vi "sub_Mock_system_IO.vi"(5 "error in":errorcluster) -> (0 "error out":errorcluster, 1 "rate":dbl=25600.0, 2 "displacement task":refnum<k21>)   [LabVIEW 2019]
uses:
  <vilib>/DAQmx/create/channels.llb/DAQmx Create Channel (AI-Voltage-Basic).vi
  <vilib>/DAQmx/configure/timing.llb/DAQmx Timing (Sample Clock).vi
  <resource>/objmgr/daqmx.rc
  <vilib>/DAQmx/write.llb/DAQmx Write (Digital 1D Bool NChan 1Samp 1Line).vi
  <vilib>/DAQmx/create/channels.llb/DAQmx Create Channel (DO-Digital Output).vi
  <vilib>/DAQmx/create/channels.llb/DAQmx Create Channel (AI-Acceleration-Accelerometer).vi
  <vilib>/DAQmx/read.llb/DAQmx Read (Analog 1D DBL 1Chan NSamp).vi
panel:
  out "time ACC Data collection":dbl
  out "acc error":errorcluster
  out "acc task":refnum<k21>
  out "Accel Data":dbl[](array[numeric])
  out "error out parker":errorcluster
  out "Parker task":refnum<k21>
  out "accelerometer sample rate (S/s)":dbl
  in  "parker error in (no error)":errorcluster caption="error in (no error)"
  in  "error in 2":errorcluster caption="error in"
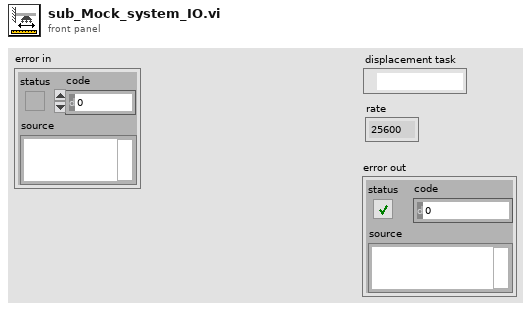
[diagram p1: front panel]
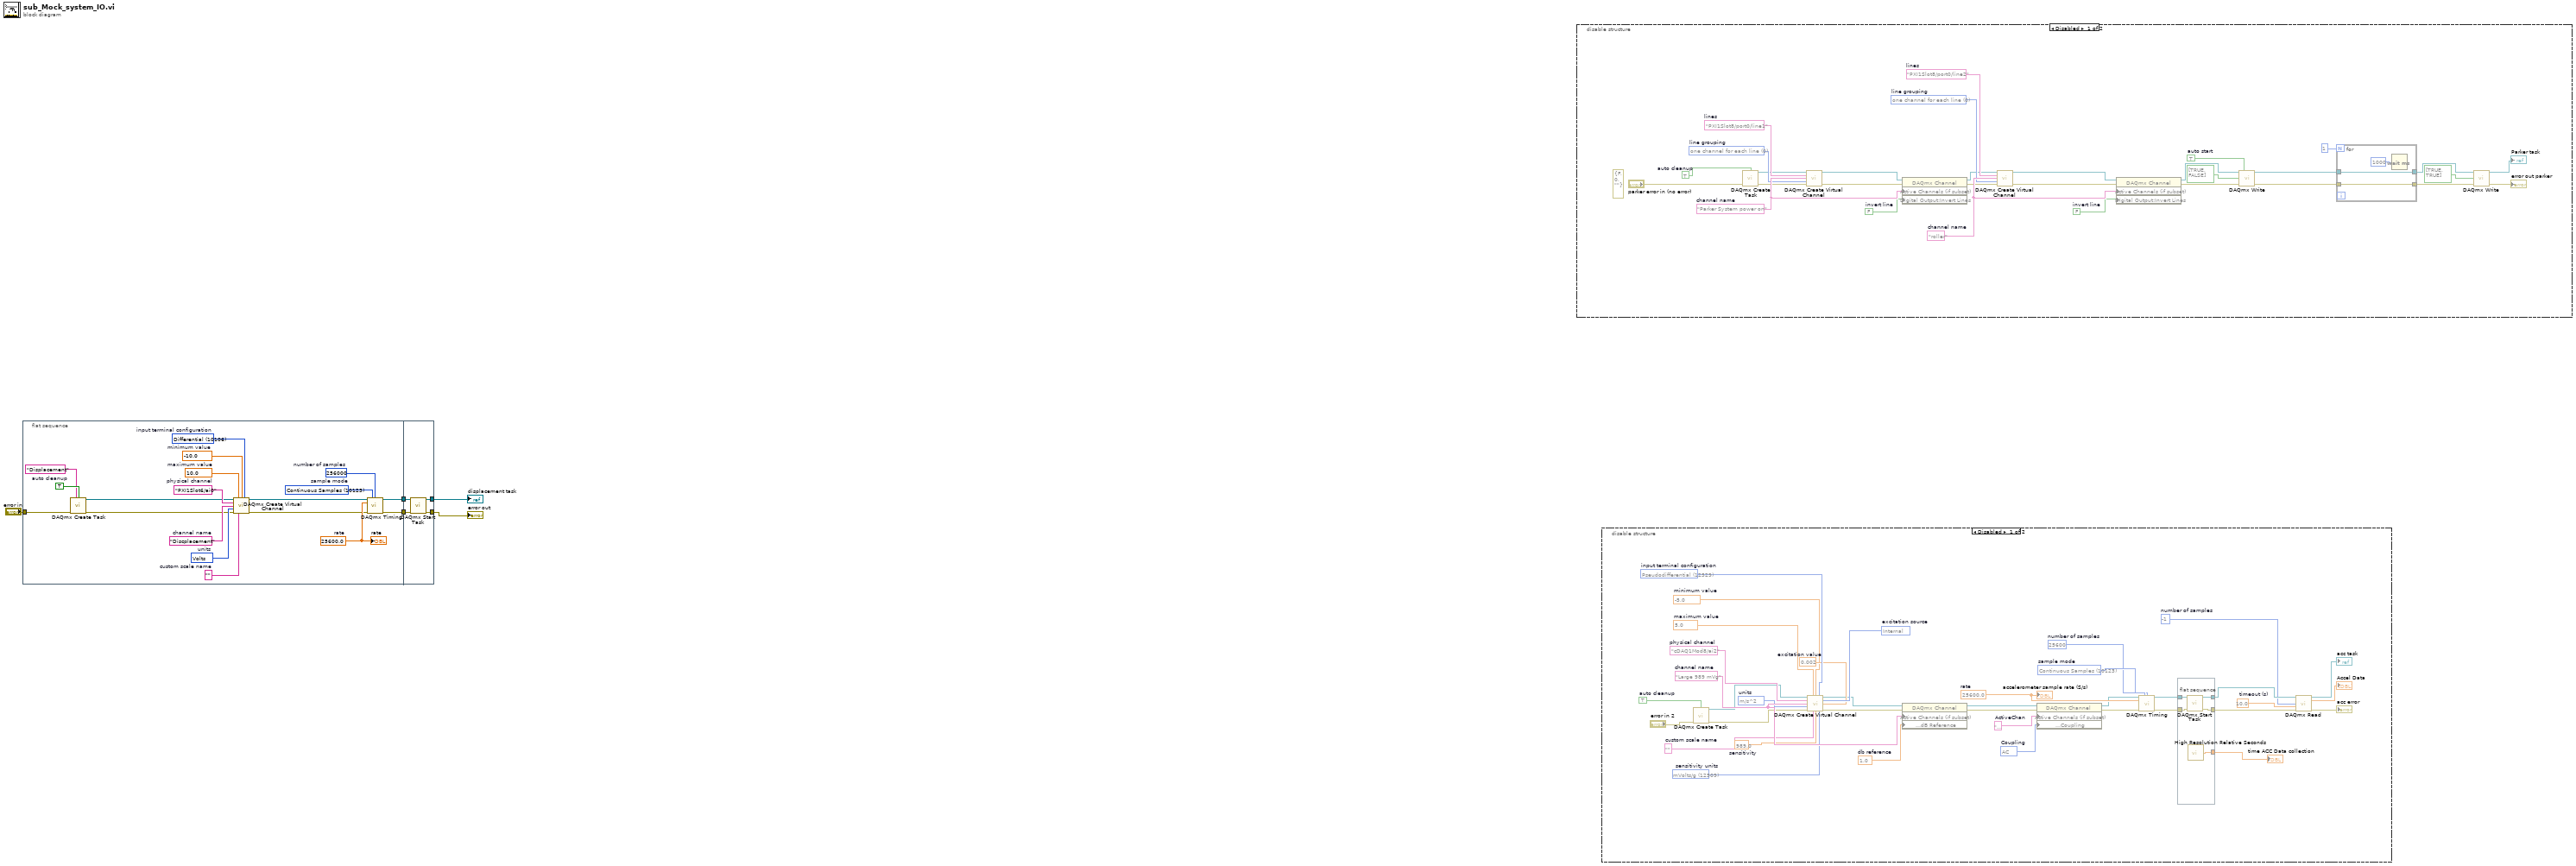
[diagram p0: block diagram]
diagram:
  n1 = flat-sequence {
    tunnel: [w8] -> w5
    tunnel: [w7] -> w4
    tunnel: "error in" -> [w9]
    tunnel: w5 -> [w27]
    tunnel: w4 -> [w28]
    tunnel: [w26] -> w3
    tunnel: [w25] -> w2
    frame #0 {
      w24 = 10123 items=["Finite Samples"=10178, "Continuous Samples"=10123, "Hardware Timed Single Point"=12522]  # sample mode
      w23 = 256000  # number of samples
      w22 = 25600.0  # rate
      w20 = 10106 items=["default"=-1, "RSE"=10083, "NRSE"=10078, "Differential"=10106, "Pseudodifferential"=12529]  # input terminal configuration
      w19 = 10348 items=["Volts"=10348, "From Custom Scale"=10065]  # units
      w18 = "Discplacement"  # channel name
      w16 = ""  # custom scale name
      w15 = -10.0  # minimum value
      w14 = 10.0  # maximum value
      w13 = "PXI1Slot6/ai0"  # physical channel
      w11 = TRUE  # auto cleanup
      n2 = call <vilib>:"DAQmx Create Task.vi"("new task name"="Displacement", "auto cleanup"=w11, "error in"=w9) -> ("task out"=w12:refnum<k21>, "error out"=w10:errorcluster)  [unwired: 11 in]
      n3 = call-poly <vilib>:"DAQmx Create Virtual Channel.vi"("task in"=w12, "maximum value"=w14, "minimum value"=w15, "input terminal configuration"=w20, "physical channels"=w13, "name to assign"=w18, "units"=w19, "error in"=w10, "custom scale name"=w16) -> ("task out"=w21:refnum<k21>, "error out"=w17:errorcluster)  [unwired: 5 in]
      n4 = call-poly <vilib>:"DAQmx Timing.vi"("task/channels in"=w21, "sample mode"=w24, "samples per channel"=w23, "rate"=w22, "error in"=w17) -> ("task out"=w7:refnum<k21>, "error out"=w8:errorcluster)  [unwired: 9 in]
      "rate" <- w22
    }
    frame #1 {
      n5 = call <vilib>:"DAQmx Start Task.vi"("task/channels in"=w28, "error in"=w27) -> ("task out"=w26:refnum<k21>, "error out"=w25:errorcluster)  [unwired: 12 in]
    }
  }
  n6 = disable-structure shown="Disabled" {
    frame Disabled {
      (unwired) errorcluster {"status"=FALSE, "code"=0, "source"=""} ("parker error in (no error)")
      w46 = FALSE  # invert line
      w43 = 0 items=["one channel for each line", "one channel for all lines"]  # line grouping
      w47 = "roller"  # channel name
      w42 = "PXI1Slot8/port0/line2"  # lines
      w39 = FALSE  # invert line
      w35 = 0 items=["one channel for each line", "one channel for all lines"]  # line grouping
      w40 = "Parker System power on"  # channel name
      w34 = "PXI1Slot8/port0/line1"  # lines
      w32 = TRUE  # auto cleanup
      w29 = TRUE  # auto start
      n7 = call <vilib>:"DAQmx Create Task.vi"("auto cleanup"=w32, "error in"="parker error in (no error)") -> ("task out"=w33:refnum<k21>, "error out"=w31:errorcluster)  [unwired: 12 in]
      n8 = call-poly <vilib>:"DAQmx Create Virtual Channel.vi"("task in"=w33, "lines"=w34, "name to assign"=w40, "line grouping"=w35, "error in"=w31) -> ("task out"=w36:refnum<k21>, "error out"=w37:errorcluster)  [unwired: 9 in]
      n9 = property class="DAQmx Channel"(reference=w36, error in=w37, "Active Channels (if subset)"=w40, "Digital Output:Invert Lines"=w39) -> (reference out=w41:refnum<k21>, error out=w38:errorcluster)
      n10 = call-poly <vilib>:"DAQmx Create Virtual Channel.vi"("task in"=w41, "lines"=w42, "name to assign"=w47, "line grouping"=w43, "error in"=w38) -> ("task out"=w44:refnum<k21>, "error out"=w45:errorcluster)  [unwired: 9 in]
      n11 = property class="DAQmx Channel"(reference=w44, error in=w45, "Active Channels (if subset)"=w47, "Digital Output:Invert Lines"=w46) -> (reference out=w48:refnum<k21>, error out=w49:errorcluster)
      n12 = call-poly <vilib>:"DAQmx Write.vi"("task/channels in"=w48, "auto start"=w29, "data"=bool[] [TRUE, FALSE], "error in"=w49) -> ("task out"=w52:refnum<k21>, "error out"=w53:errorcluster)  [unwired: 9 in, 1 out]
      n13 = for {
        N: 1 -> [_]
        tunnel: [w61] -> w51
        tunnel: w52 -> [w61]
        tunnel: w53 -> [w60]
        tunnel: [w60] -> w54
        n14 = Wait (ms)(milliseconds to wait=u32 1000) -> ()  [unwired: 1 out]
      }
      n15 = call-poly <vilib>:"DAQmx Write.vi"("task/channels in"=w51, "data"=bool[] [TRUE, TRUE], "error in"=w54) -> ("task out"=→"Parker task":refnum<k21>, "error out"=→"error out parker":errorcluster)  [unwired: 10 in, 1 out]
    }
    frame Enabled {
    }
  }
  n16 = disable-structure shown="Disabled" {
    frame Disabled {
      w92 = 10.0  # timeout (s)
      w91 = -1  # number of samples
      w88 = 10123 items=["Finite Samples"=10178, "Continuous Samples"=10123, "Hardware Timed Single Point"=12522]  # sample mode
      w87 = 25600  # number of samples
      w98 = 25600.0  # rate
      w83 = 10045 items=["AC"=10045, "DC"=10050, "GND"=10066]  # Coupling
      w82 = "Large 989 mVg"  # ActiveChan
      w80 = 1.0  # db reference
      w77 = 12470 items=["g"=10186, "m/s^2"=12470, "From Custom Scale"=10065]  # units
      w76 = 12529 items=["default"=-1, "RSE"=10083, "NRSE"=10078, "Differential"=10106, "Pseudodifferential"=12529]  # input terminal configuration
      w75 = 10200 items=["Internal"=10200, "External"=10167, "None"=10230]  # excitation source
      w74 = 0.002  # excitation value
      w73 = 12509 items=["mVolts/g"=12509, "Volts/g"=12510]  # sensitivity units
      w72 = 989.0  # sensitivity
      w81 = "Large 989 mVg"  # channel name
      w70 = ""  # custom scale name
      w69 = -5.0  # minimum value
      w68 = 5.0  # maximum value
      w67 = "cDAQ1Mod8/ai2"  # physical channel
      w65 = TRUE  # auto cleanup
      n17 = call <vilib>:"DAQmx Create Task.vi"("auto cleanup"=w65, "error in"="error in 2") -> ("task out"=w66:refnum<k21>, "error out"=w64:errorcluster)  [unwired: 12 in]
      n18 = call-poly <vilib>:"DAQmx Create Virtual Channel.vi"("task in"=w66, "maximum value"=w68, "minimum value"=w69, "input terminal configuration"=w76, "physical channels"=w67, "current excitation source"=w75, "name to assign"=w81, "current excitation value"=w74, "units"=w77, "error in"=w64, "custom scale name"=w70, "sensitivity"=w72, "sensitivity units"=w73) -> ("task out"=w71:refnum<k21>, "error out"=w78:errorcluster)  [unwired: 1 in]
      n19 = property class="DAQmx Channel"(reference=w71, error in=w78, "Active Channels (if subset)"=w81, "Analog Input:Acceleration:dB Reference"=w80) -> (reference out=w85:refnum<k21>, error out=w79:errorcluster)
      n20 = property class="DAQmx Channel"(reference=w85, error in=w79, "Active Channels (if subset)"=w82, "Analog Input:General Properties:Input Configuration:Coupling"=w83) -> (reference out=w86:refnum<k21>, error out=w84:errorcluster)
      n21 = call-poly <vilib>:"DAQmx Timing.vi"("task/channels in"=w86, "sample mode"=w88, "samples per channel"=w87, "rate"=w98, "error in"=w84) -> ("task out"=w89:refnum<k21>, "error out"=w90:errorcluster)  [unwired: 9 in]
      n22 = flat-sequence {
        tunnel: [w103] -> w95
        tunnel: [w102] -> w93
        tunnel: w90 -> [w101]
        tunnel: w89 -> [w100]
        tunnel: [w99] -> w62
        frame #0 {
          n23 = call <vilib>:"DAQmx Start Task.vi"("task/channels in"=w100, "error in"=w101) -> ("task out"=w103:refnum<k21>, "error out"=w102:errorcluster)  [unwired: 12 in]
          n24 = call <vilib>:"High Resolution Relative Seconds.vi"() -> ("relative seconds"=w99:dbl)
        }
      }
      n25 = call-poly <vilib>:"DAQmx Read.vi"("task/channels in"=w95, "number of samples per channel"=w91, "timeout"=w92, "error in"=w93) -> ("task out"=→"acc task":refnum<k21>, "data"=→"Accel Data":dbl[], "error out"=→"acc error":errorcluster)  [unwired: 9 in]
      "accelerometer sample rate (S/s)" <- w98
      "time ACC Data collection" <- w62
    }
    frame Enabled {
    }
  }
  "error out" <- w2
  "displacement task" <- w3
